vi "GVmotor_convert_step_vs_turn.vi"(7 "backlash_corr":bool=TRUE caption="Backlash Correction", 8 "turn_in_pre":dbl, 9 "turn_in":dbl, 10 "step_in_pre":i32, 11 "step_in":i32) -> (0 "step_corr_for_step_out":i32, 1 "step_out":i32, 2 "step_corr_for_turn_out":i32, 3 "turn_out":dbl, 4 "step_change_sign":i8)   [LabVIEW 2019]
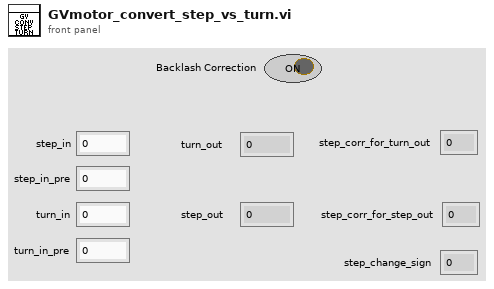
[diagram p1: front panel]
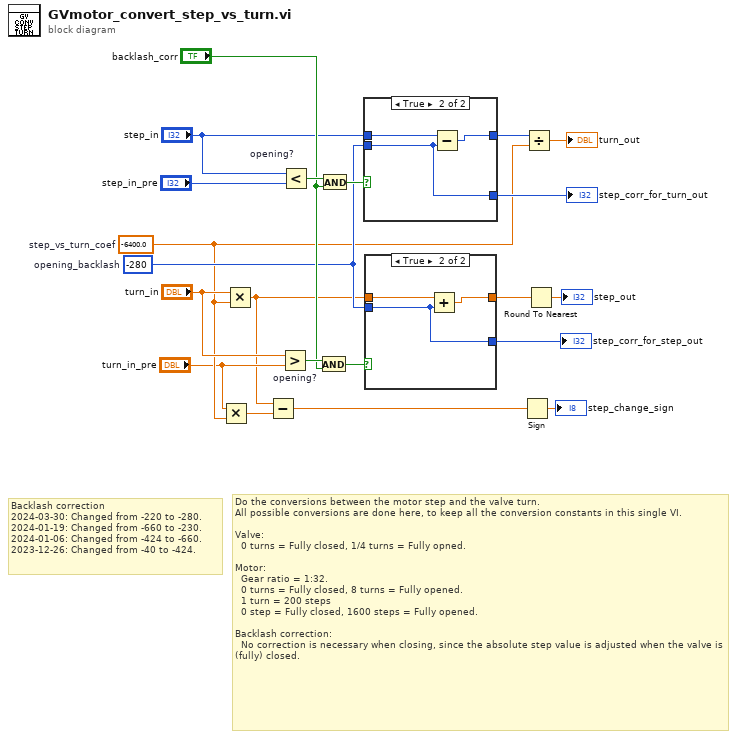
[diagram p0: block diagram]
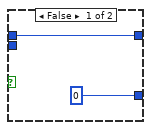
[diagram p2: hidden frame]
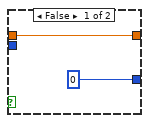
[diagram p3: hidden frame]
diagram:
  w9 = -280  # opening_backlash
  w6 = -6400.0  # step_vs_turn_coef
  # "Backlash correction\n2024-03-30: Changed from -220 to -280.\n2024-01-19: Changed from -660 to -230.\n2024-01-06: Changed from -424 to -660.\n2023-12-26: Changed from -40 to -424."
  # "Do the conversions between the motor step and the valve turn.\nAll possible conversions are done here, to keep all the conversion constants in this single VI.\n\nValve: \n  0 turns = Fully closed, 1/4 turns = Fully opned.\n\nMotor: \n  Gear ratio = 1:32.\n  0 turns = Fully closed, 8 turns = Fully opened.\n  1 turn = 200 steps\n  0 step = Fully closed, 1600 steps = Fully opened.\n\nBacklash correction:\n  No correction is necessary when closing, since the absolute step value is adjusted when the valve is (fully) closed."
  n1 = Multiply(x="turn_in_pre", y=w6) -> (x*y=w4:dbl)
  n2 = Multiply(x="turn_in", y=w6) -> (x*y=w3:dbl)
  n3 = Subtract(x=w3, y=w4) -> (x-y=w1:dbl)
  n4 = Greater? "opening?"(x="turn_in", y="turn_in_pre") -> (0:w18:bool)
  n5 = Less? "opening?"(x="step_in", y="step_in_pre") -> (x < y?=w14:bool)
  n6 = And(x=w18, y="backlash_corr") -> (x .and. y?=w17:bool)
  n7 = And(x=w14, y="backlash_corr") -> (x .and. y?=w12:bool)
  n8 = case shown="True" w12 {
    tunnel: [w23 w25] -> w11
    tunnel: "step_in" -> [w23 w26]
    tunnel: w9 -> [_ w24]
    tunnel: [0 ("opening_backlash") w24] -> w7
    frame False {
    }
    frame True {
      n9 = Subtract(x=w26, y=w24) -> (x-y=w25:i32)
    }
  }
  "step_corr_for_turn_out" <- w7
  n10 = case shown="True" w17 {
    tunnel: w3 -> [w28 w30]
    tunnel: [w28 w31] -> w16
    tunnel: [0 ("step_corr") w29] -> w8
    tunnel: w9 -> [_ w29]
    frame False {
    }
    frame True {
      n11 = Add(x=w30, y=w29) -> (x+y=w31:dbl)
    }
  }
  "step_corr_for_step_out" <- w8
  n12 = Sign(1:w1) -> (0:→"step_change_sign":dbl)
  n13 = Divide(x=w11, y=w6) -> (x/y=→"turn_out":dbl)
  n14 = Round To Nearest(number=w16) -> (nearest integer value=→"step_out":dbl)
